vi "zmq_z85_encode.vi"(3 "error in":errorcluster, 4 "zero pad? (F)":bool, 5 "data in":u8[](array[numeric])) -> (0 "error out":errorcluster, 2 "encoded string":string)   [LabVIEW 2020, in "zeromq.lvlib"]
doc: "Queries and returns the version of ZeroMQ currently loaded as both a string and struct.\n\nDetailed API documentation: http://api.zeromq.org/3-2:zmq-version"
uses:
  zeromq.lvlib
panel:
  # "ØMQ"
  # "labview"
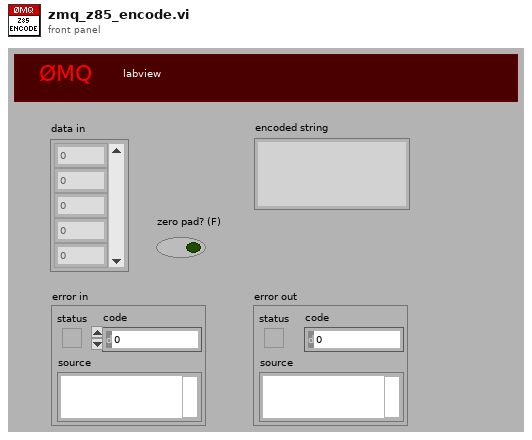
[diagram p1: front panel]
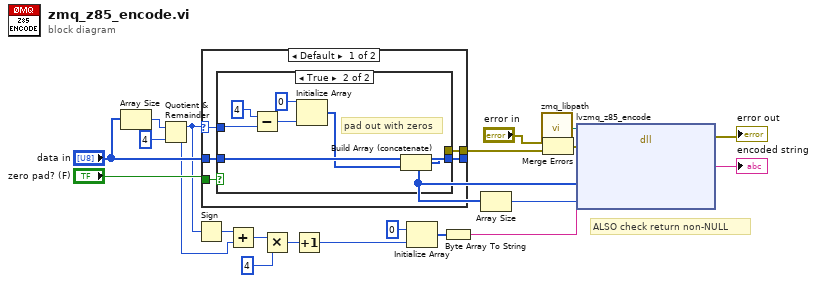
[diagram p0: block diagram]
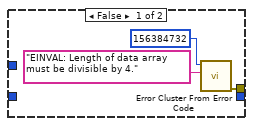
[diagram p2: hidden frame]
diagram:
  # "ALSO check return non-NULL"
  n1 = Array Size(array="data in") -> (size(s)=w7:i32)
  n2 = Quotient & Remainder(x=w7, y=4) -> (x-y*floor(x/y)=w6:i32, floor(x/y)=w4:i32)
  n3 = Sign(1:w6) -> (0:w5:i32)
  n4 = case shown="Default" w6 {
    selector: w6 -> [w25 _]
    tunnel: "zero pad? (F)" -> [w27 _]
    tunnel: "data in" -> [w26 w38]
    tunnel: [w24 w38] -> w16
    tunnel: [w23 _] -> w12
    frame Default {
      n5 = case shown="True" w27 {
        tunnel: w26 -> [_ w35]
        tunnel: w25 -> [_ w37]
        tunnel: [_ w31] -> w24
        tunnel: [w28 _] -> w23
        frame False {
          n6 = call "Error Cluster From Error Code.vi"("error message (\"\")"="EINVAL: Length of data array must be divisible by 4." ("error message (\"\")"), "error code (0)"=156384732) -> ("error out"=w28:errorcluster)  [unwired: 7 in]
        }
        frame True {
          # "pad out with zeros"
          n7 = Subtract(x=4 ("y"), y=w37) -> (x-y=w34:i32)
          n8 = Initialize Array(u8 0 ("element"), w34) -> (w32:u8[])
          n9 = Build Array (concatenate)(w35, w32) -> (w31:u8[])
        }
      }
    }
    frame 0 {
      # "Divisible by 4, is ok"
    }
  }
  n10 = Add(x=w5, y=w4) -> (x+y=w3:i32)
  n11 = Multiply(x=w3, y=4) -> (x*y=w1:i32)
  n12 = Increment(x=w1) -> (x+1=w9:i32)
  n13 = Initialize Array(u8 0 ("element"), w9) -> (w11:u8[])
  n14 = Byte Array To String(unsigned byte array=w11) -> (string=w10:string)
  n15 = Array Size(array=w16) -> (size(s)=w15:i32)
  n16 = call "zmq_libpath.vi"() -> ("path"=w21:path)
  n17 = Merge Errors("error in", w12) -> (w14:errorcluster)
  n18 = dll-call lib="?" fn="lvzmq_z85_encode" ("zmq_labview.dll:lvzmq_socket")(path in=w21, error in=w14, "dest"=w10, "src"=w16, "len"=w15) -> (error out=→"error out":errorcluster, "dest"=→"encoded string":string)  [unwired: 4 in, 1 out]
